vi "Test_IncrementValuePublication_DBL_ValueIncremented.vi"(8 "error in (no error)":errorcluster, 11 "TestCase in":refnum<class "TestPublicationPolicy.lvclass">) -> (0 "error out":errorcluster, 3 "TestCase out":refnum<class "TestPublicationPolicy.lvclass">)   [LabVIEW 2017, in "TestPublicationPolicy.lvclass"]
uses:
  TestPublicationPolicy.lvclass
  Source/Framework/PublicationPolicy/IncrementValuePublication/IncrementValuePublication.lvclass
  C:/Git/mva-framework/Source/Framework/IMediator/IPublicationPolicy/IPublicationPolicy.lvclass
  Source/Framework/IMediator/IPublicationPolicy/IPublicationPolicy.lvclass
  gpm_packages/@cs/transport/Source/Concrete/NotifierTransport/NotifierTransport.lvclass/NotifierTransport.ctl
  Source/Framework/IMediator/PublishRequest/PublishRequest.lvclass/PublishRequest.ctl
  Source/Framework/IMediator/MutexedPublishRequest/MutexedPublishRequest.lvclass/MutexedPublishRequest.ctl
  Source/Framework/IMediator/PublishRequest/Write Publish Request Data.vi
  gpm_packages/@cs/transport/Source/Concrete/NotifierTransport/NotifierTransport.lvclass
  C:/Git/mva-framework/gpm_packages/@cs/transport/Source/ITransport/ITransport.lvclass
  Source/Framework/IMediator/MutexedPublishRequest/MutexedPublishRequest.lvclass
  C:/Git/mva-framework/Source/Framework/IMediator/PublishRequest/PublishRequest.lvclass
  <vilib>/Utility/error.llb/Error Cluster From Error Code.vi
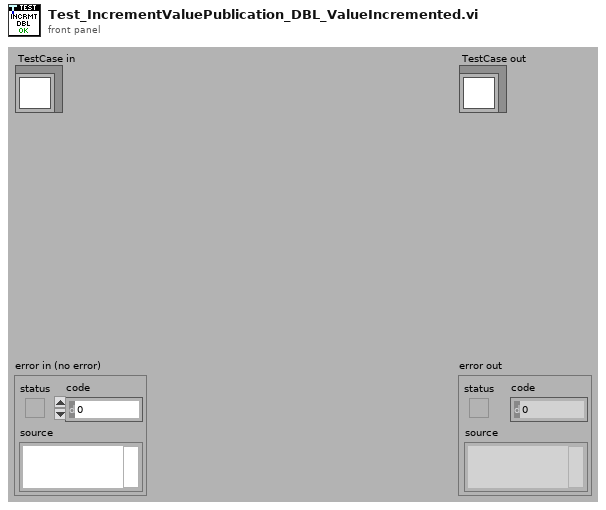
[diagram p1: front panel]
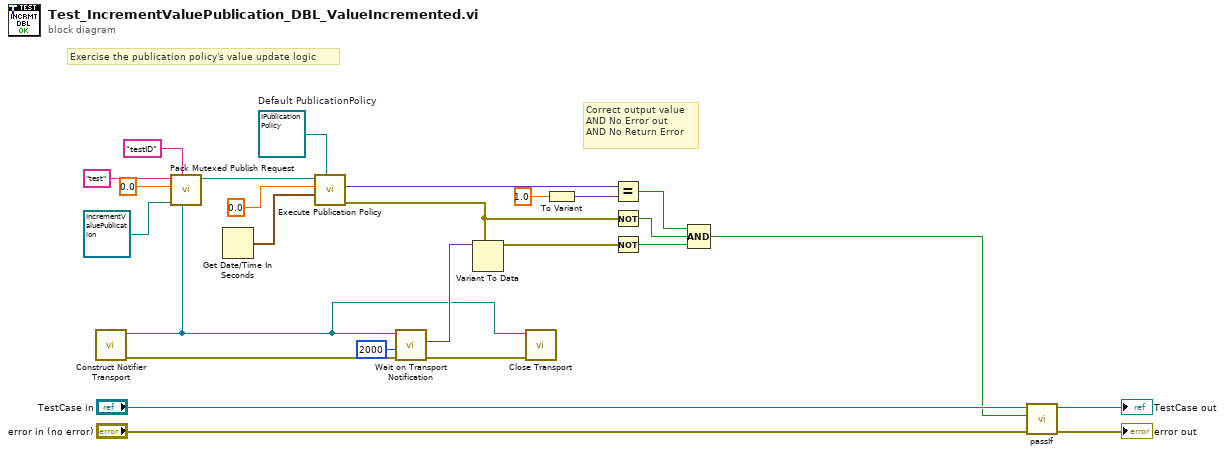
[diagram p0: block diagram]
diagram:
  w18 = refnum<class "IPublicationPolicy.lvclass"> refnum  # Default PublicationPolicy
  # "Correct output value\nAND No Error out\nAND No Return Error"
  # "Exercise the publication policy's value update logic"
  n1 = call "Construct Notifier Transport.vi"() -> ("error out"=w14:errorcluster, "NotifierTransport"=w2:refnum<class "NotifierTransport.lvclass">)  [unwired: 10 in]
  n2 = call "Pack Mutexed Publish Request.vi"("Return Error Transport"=w2, "Publisher ID"="testID", "PublicationPolicy"=refnum<class "IncrementValuePublication.lvclass"> refnum ("PublicationPolicy.lvlib:IncrementValuePublication.lvclass"), "Datum Value or Type"=0.0 ("Data to Publish"), "Datum Name"="test") -> ("MutexedPublishRequest Out"=w20:refnum<class "MutexedPublishRequest.lvclass">)  [unwired: 6 in]
  n3 = Get Date/Time In Seconds() -> (seconds since 1Jan1904=w21:timestamp)
  n4 = call-dynamic "Execute Publication Policy.vi"("Default PublicationPolicy"=w18, "Last Publish Time"=w21, "Last Published Value"=0.0, "MutexedPublishRequest"=w20) -> ("error out (Reject Publication)"=w4:errorcluster, "Value to Publish"=w11:variant)  [unwired: 5 in, 1 out]
  n5 = call "Wait on Transport Notification.vi"("error in (no error)"=w14, "Timeout In ms (-1)"=2000, "NotifierTransport"=w2) -> ("error out"=w1:errorcluster, "Data"=w12:variant)  [unwired: 6 in, 1 out]
  n6 = Variant To Data(type=w4, Variant=w12) -> (data=w8:errorcluster)  [unwired: 1 in, 1 out]
  n7 = call-dynamic "Close Transport.vi"("error in (no error)"=w1, "NotifierTransport"=w2) -> ()  [unwired: 9 in, 1 out]
  n8 = To Variant(anything=1.0) -> (Variant=w9:variant)
  n9 = Equal?(x=w11, y=w9) -> (x = y?=w7:bool)
  n10 = Not(x=w4) -> (.not. x?=w3:bool)
  n11 = Not(x=w8) -> (.not. x?=w5:bool)
  n12 = Compound Arithmetic op=AND(w7, w3, w5) -> (w6:bool)
  n13 = call-dynamic "passIf.vi"("error in (no error)"="error in (no error)", "pass"=w6, "TestCase in"="TestCase in") -> ("error out"=→"error out":errorcluster, "TestCase out"=→"TestCase out":refnum<class "TestPublicationPolicy.lvclass">)  [unwired: 7 in]
